vi "Sequence.BuildPreviewWaveform.vi"(7 "WaveformGraph in":refnum<vi>, 8 "error in (no error)":errorcluster, 9 "Rows":cluster{"Start Index":i32, "Length":i32}={"Start Index"=0, "Length"=-1}, 10 "UI.Sequence#ofColumns":i32, 11 "SequenceRef":refnum<vi>) -> (0 "error out":errorcluster, 2 "Wavefrom":waveform(dbl)[](array[waveform]))   [LabVIEW 2013, in "Simple Sequence Tools - Shared.lvlib"]
uses:
  Simple Sequence Tools - Shared.lvlib
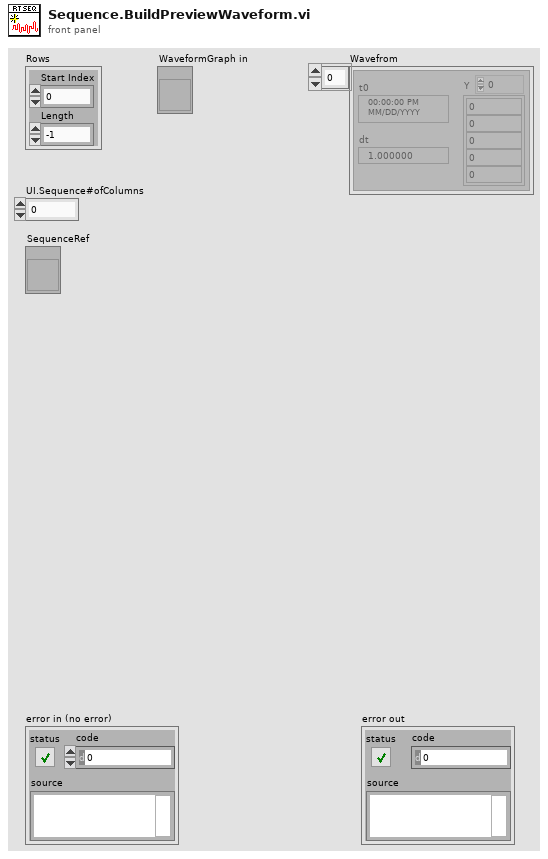
[diagram p1: front panel]
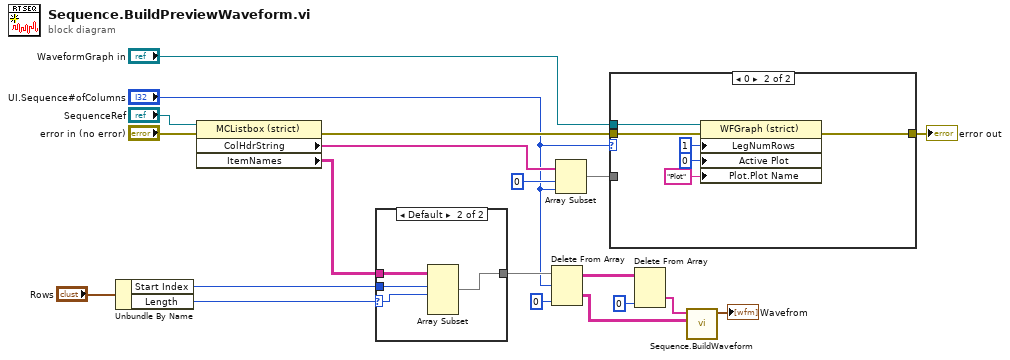
[diagram p0: block diagram]
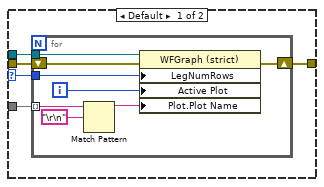
[diagram p2: hidden frame]
diagram:
  n1 = Unbundle By Name("Rows") -> ("Start Index"=w5:i32, "Length"=w8:i32)
  n2 = property class="MCListbox (strict)"(reference="SequenceRef", error in="error in (no error)") -> (error out=w10:errorcluster, "ColHdrString"=w12:string[], "ItemNames"=w7:string[][])  [unwired: 1 out]
  n3 = case shown="Default" w8 {
    selector: w8 -> [_ w22]
    tunnel: w7 -> [w21 w25]
    tunnel: [w21 w24] -> w6
    tunnel: w5 -> [_ w23]
    frame -1 {
    }
    frame Default {
      n4 = Array Subset(array=w25, index (row)=w23, length (row)=w22) -> (w24:string[][])  [unwired: 2 in]
    }
  }
  n5 = Delete From Array(array=w6, length="UI.Sequence#ofColumns", index (col)=0 ("disabled index (col)")) -> (deleted portion=w4:string[][], array with subset deleted=w16:string[][])  [unwired: 1 in]
  n6 = Array Subset(array=w12, index=0, length="UI.Sequence#ofColumns") -> (w19:string[])
  n7 = case shown="0" "UI.Sequence#ofColumns" {
    selector: "UI.Sequence#ofColumns" -> [w26 _]
    tunnel: [w30 w44] -> w20
    tunnel: w19 -> [w29 _]
    tunnel: "WaveformGraph in" -> [w28 w43]
    tunnel: w10 -> [w27 w42]
    frame Default {
      n8 = for {
        tunnel: w26 -> [w38]
        tunnel: w29 -> [w35] mode=indexing
        shift-right: [w32] -> w30
        shift-left: w27 -> [w33]
        tunnel: w28 -> [w31]
        i -> [w37]
        n9 = Match Pattern(string=w35, regular expression="\r\n") -> (before substring=w36:string)  [unwired: 1 in, 3 out]
        n10 = property on="Property Node" class="WFGraph (strict)"(reference=w31, error in=w33, "LegNumRows"=w38, "Active Plot"=w37, "Plot.Plot Name"=w36) -> (error out=w32:errorcluster)  [unwired: 1 out]
      }
    }
    frame 0 {
      n11 = property on="Property Node" class="WFGraph (strict)"(reference=w43, error in=w42, "LegNumRows"=u32 1 ("Legend:Number of Rows"), "Active Plot"=u32 0, "Plot.Plot Name"="Plot") -> (error out=w44:errorcluster)  [unwired: 1 out]
    }
  }
  "error out" <- w20
  n12 = Delete From Array(array=w16, index (col)=0 ("disabled index (col)")) -> (deleted portion=w3:string[])  [unwired: 2 in, 1 out]
  n13 = call "Sequence.BuildWaveform.vi"("Steps"=w4, "Duration"=w3) -> ("Array"=→"Wavefrom":waveform(dbl)[])  [unwired: 9 in]
